vi "MotionController.vi"() -> (0 "error out":errorcluster)   [LabVIEW 2017]
uses:
  MCTypedef.ctl
  <vilib>/Instr/_visa.llb/VISA Configure Serial Port (Instr).vi
  <vilib>/Utility/inputDevices.llb/keyboardAcquire.vi
panel:
  in  "sp33d":dbl(knob)=0.5 step=0.5 scale=0.5..1.0
  in  "clear":bool
  out "read buffer":string
  in  "End Program":bool
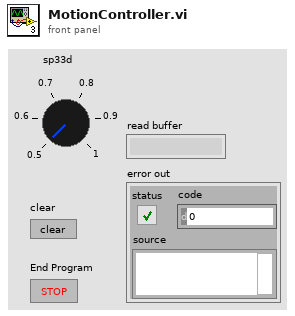
[diagram p1: front panel]
types:
  T1 = typedef "MCTypedef.ctl" = enum16{"idle", "forward", "reverse", "clear"}
  T2 = enum16{"0", "1", "2", "3", "4", "5", "6", "7", "8", "9", "A", "B", "C", "D", "E", "F", "G", "H", "I", "J", "K", "L", "M", "N", "O", "P", "Q", "R", "S", "T", "U", "V", "W", "X", "Y", "Z", "F1", "F2", "F3", "F4", "F5", "F6", "F7", "F8", "F9", "F10", "F11", "F12", "F13", "F14", "F15", "ADD", "BACK", "BACKSLASH", "CAPITAL", "COMMA", "DECIMAL", "DELETE", "DIVIDE", "DOWN", "END", "EQUALS", "ESCAPE", "GRAVE (`)", "HOME", "INSERT", "LBRACKET", "LCONTROL", "LEFT", "L ALT", "LSHIFT", "LWIN", "MINUS", "MULTIPLY", "NEXT", "NUMLOCK", "NUMPAD_0", "NUMPAD_1", "NUMPAD_2", "NUMPAD_3", "NUMPAD_4", "NUMPAD_5", "NUMPAD_6", "NUMPAD_7", "NUMPAD_8", "NUMPAD_9", "PAUSE", "PERIOD", "PRIOR (PG UP)", "RBRACKET", "RCONTROL", "RETURN", "RIGHT", "R ALT", "RSHIFT", "RWIN", "SCROLL", "SEMICOLON", "SLASH", "SPACE", "SUBTRACT", "TAB", "UP", "ENTER (num pad)", "' (quote)"}[]
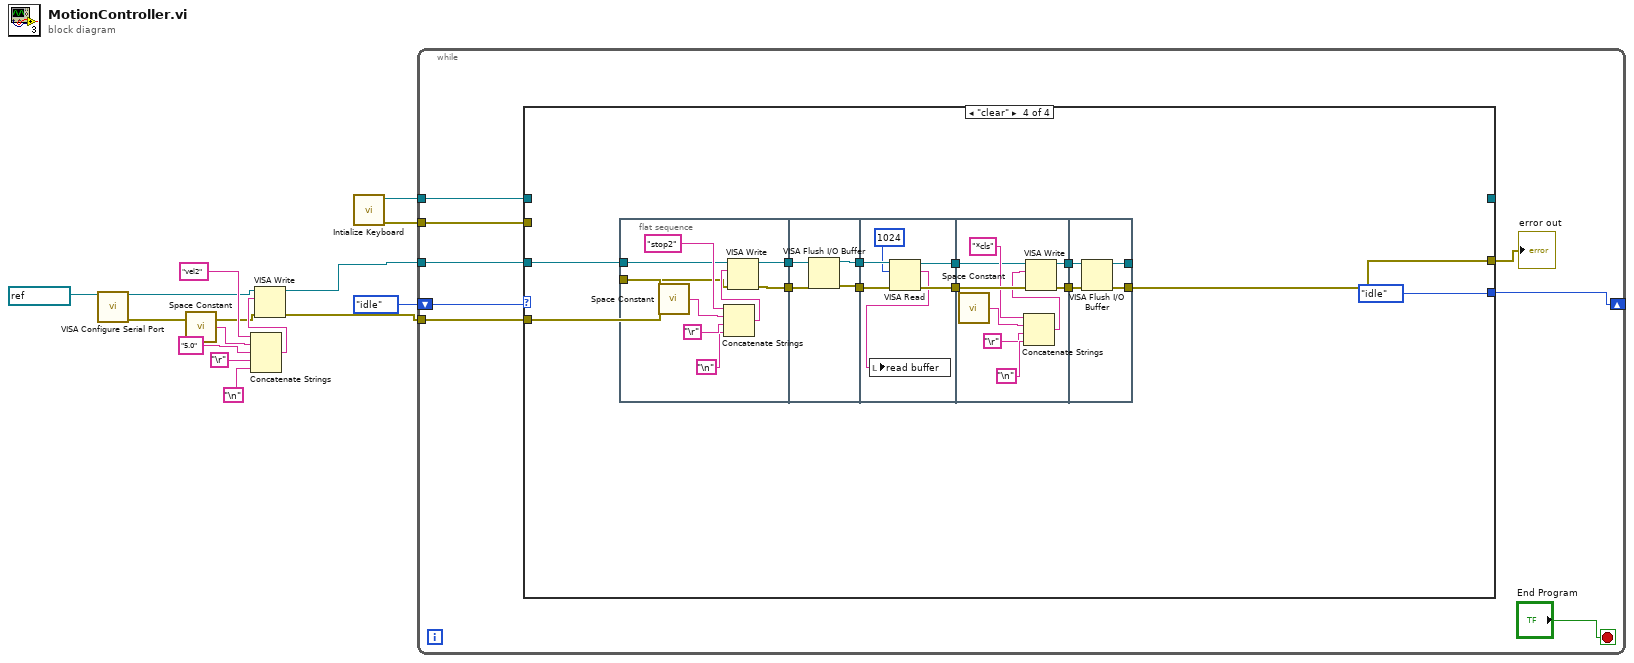
[diagram p0: block diagram]
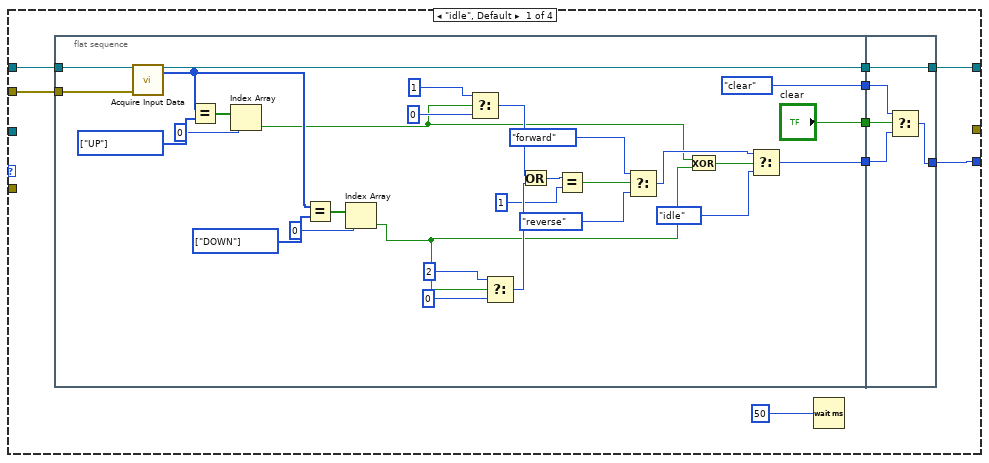
[diagram p2: hidden frame]
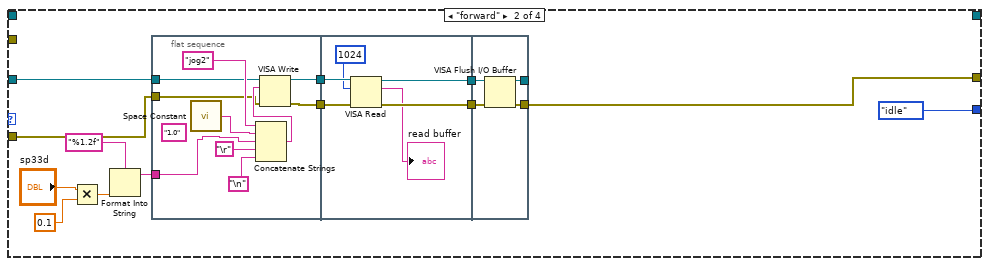
[diagram p3: hidden frame]
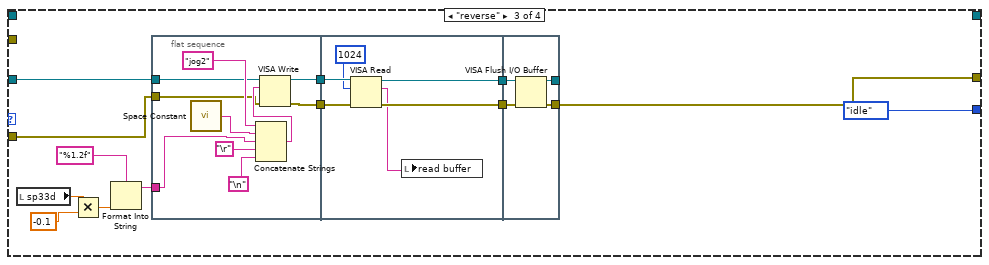
[diagram p4: hidden frame]
diagram:
  n1 = call-poly "VISA Configure Serial Port"("VISA resource name"=refnum<visa-resource-name> "COM1") -> ("VISA resource name out"=w5:refnum<visa-resource-name>, "error out"=w4:errorcluster)  [unwired: 13 in]
  n2 = call <vilib>:"Space Constant.vi"() -> ("String"=w11:string)
  n3 = Concatenate Strings("vel2" ("string"), w11, "5.0" ("string"), "\r", "\n") -> (w10:string)
  n4 = VISA Write(VISA resource name=w5, write buffer=w10, error in (no error)=w4) -> (VISA resource name out=w3:refnum<visa-resource-name>, error out=w2:errorcluster)  [unwired: 1 out]
  n5 = call <vilib>:"Intialize Keyboard.vi"() -> ("error out"=w12:errorcluster, "device ID"=w13:refnum<k1>)  [unwired: 10 in]
  n6 = while {
    shift-right: [w21] -> _
    shift-left: MCTypedef."idle" -> [w22]
    tunnel: w3 -> [w18]
    tunnel: w2 -> [w17]
    tunnel: w13 -> [w16]
    tunnel: w12 -> [w15]
    stop <- "End Program" stop-if-true
    n7 = case shown="\"clear\"" w22 {
      tunnel: [w23 MCTypedef."idle" MCTypedef."idle" MCTypedef."idle"] -> w21
      tunnel: [_ w73 w106 w142] -> w19
      tunnel: w18 -> [_ w72 w105 w141]
      tunnel: w17 -> [_ w71 w104 w140]
      tunnel: w16 -> [w30 _ _ _]
      tunnel: w15 -> [w28 _ _ _]
      tunnel: [w29 _ _ _] -> _
      frame "idle", Default {
        n8 = flat-sequence {
          tunnel: w30 -> [w46]
          tunnel: w28 -> [w41]
          tunnel: [w45] -> w27
          tunnel: [MCTypedef."clear" ("t")] -> w26
          tunnel: ["clear"] -> w25
          tunnel: [w32] -> w24
          tunnel: [w65] -> w29
          tunnel: w27 -> [w65]
          tunnel: w26 -> [w63]
          tunnel: w25 -> [w64]
          tunnel: w24 -> [w62]
          tunnel: [w61] -> w23
          frame #0 {
            w38 = T2 [enum."DOWN"] items=["0", "1", "2", "3", "4", "5", "6", "7", "8", "9", "A", "B", "C", "D", "E", "F", "G", "H", "I", "J", "K", "L", "M", "N", "O", "P", "Q", "R", "S", "T", "U", "V", "W", "X", "Y", "Z", "F1", "F2", "F3", "F4", "F5", "F6", "F7", "F8", "F9", "F10", "F11", "F12", "F13", "F14", "F15", "ADD", "BACK", "BACKSLASH", "CAPITAL", "COMMA", "DECIMAL", "DELETE", "DIVIDE", "DOWN", "END", "EQUALS", "ESCAPE", "GRAVE (`)", "HOME", "INSERT", "LBRACKET", "LCONTROL", "LEFT", "L ALT", "LSHIFT", "LWIN", "MINUS", "MULTIPLY", "NEXT", "NUMLOCK", "NUMPAD_0", "NUMPAD_1", "NUMPAD_2", "NUMPAD_3", "NUMPAD_4", "NUMPAD_5", "NUMPAD_6", "NUMPAD_7", "NUMPAD_8", "NUMPAD_9", "PAUSE", "PERIOD", "PRIOR (PG UP)", "RBRACKET", "RCONTROL", "RETURN", "RIGHT", "R ALT", "RSHIFT", "RWIN", "SCROLL", "SEMICOLON", "SLASH", "SPACE", "SUBTRACT", "TAB", "UP", "ENTER (num pad)", "' (quote)"] ("y")
            w44 = T2 [enum."UP"] items=["0", "1", "2", "3", "4", "5", "6", "7", "8", "9", "A", "B", "C", "D", "E", "F", "G", "H", "I", "J", "K", "L", "M", "N", "O", "P", "Q", "R", "S", "T", "U", "V", "W", "X", "Y", "Z", "F1", "F2", "F3", "F4", "F5", "F6", "F7", "F8", "F9", "F10", "F11", "F12", "F13", "F14", "F15", "ADD", "BACK", "BACKSLASH", "CAPITAL", "COMMA", "DECIMAL", "DELETE", "DIVIDE", "DOWN", "END", "EQUALS", "ESCAPE", "GRAVE (`)", "HOME", "INSERT", "LBRACKET", "LCONTROL", "LEFT", "L ALT", "LSHIFT", "LWIN", "MINUS", "MULTIPLY", "NEXT", "NUMLOCK", "NUMPAD_0", "NUMPAD_1", "NUMPAD_2", "NUMPAD_3", "NUMPAD_4", "NUMPAD_5", "NUMPAD_6", "NUMPAD_7", "NUMPAD_8", "NUMPAD_9", "PAUSE", "PERIOD", "PRIOR (PG UP)", "RBRACKET", "RCONTROL", "RETURN", "RIGHT", "R ALT", "RSHIFT", "RWIN", "SCROLL", "SEMICOLON", "SLASH", "SPACE", "SUBTRACT", "TAB", "UP", "ENTER (num pad)", "' (quote)"] ("y")
            n9 = call-poly <vilib>:"Acquire Input Data.vi"("device ID"=w46, "error in (no error)"=w41) -> ("device ID"=w45:refnum<k1>, "keys pressed"=w37:T2)  [unwired: 15 in, 1 out]
            n10 = Equal?(x=w37, y=w44) -> (x = y?=w43:bool[])
            n11 = Index Array(array=w43, index=0) -> (element=w36:bool)
            n12 = Equal?(x=w37, y=w38) -> (x = y?=w39:bool[])
            n13 = Index Array(array=w39, index=0) -> (element=w35:bool)
            n14 = Select(t=1, s=w36, f=0) -> (s? t:f=w55:i32)
            n15 = Select(t=2, s=w35, f=0) -> (s? t:f=w54:i32)
            n16 = Or(x=w55, y=w54) -> (x .or. y?=w53:i32)
            n17 = Equal?(x=w53, y=1) -> (x = y?=w51:bool)
            n18 = Select(t=MCTypedef."forward", s=w51, f=MCTypedef."reverse") -> (s? t:f=w47:T1)
            n19 = Exclusive Or(1:w35, 2:w36) -> (0:w60:bool)
            n20 = Select(t=w47, s=w60, f=MCTypedef."idle") -> (s? t:f=w32:T1)
          }
          frame #1 {
            n21 = Select(t=w63, s=w64, f=w62) -> (s? t:f=w61:T1)
          }
        }
        n22 = Wait (ms)(milliseconds to wait=u32 50) -> ()  [unwired: 1 out]
      }
      frame "forward" {
        n23 = Multiply(x="sp33d", y=0.1) -> (x*y=w68:dbl)
        n24 = Format Into String(format string="%1.2f", w68) -> (resulting string=w66:string)  [unwired: 2 in, 1 out]
        n25 = flat-sequence {
          tunnel: [w88] -> w78
          tunnel: [w87] -> w77
          tunnel: w72 -> [w81]
          tunnel: w71 -> [w80]
          tunnel: w66 -> [w79]
          tunnel: w78 -> [w94]
          tunnel: w77 -> [w93]
          tunnel: [w92] -> w76
          tunnel: [w91] -> w75
          tunnel: w76 -> [w97]
          tunnel: w75 -> [w98]
          tunnel: [w96] -> _
          tunnel: [w95] -> w73
          frame #0 {
            (unwired) "1.0" ("string")
            n26 = call <vilib>:"Space Constant.vi"() -> ("String"=w82:string)
            n27 = Concatenate Strings("jog2" ("string"), w82, w79, "\r", "\n") -> (w83:string)
            n28 = VISA Write(VISA resource name=w81, write buffer=w83, error in (no error)=w80) -> (VISA resource name out=w88:refnum<visa-resource-name>, error out=w87:errorcluster)  [unwired: 1 out]
          }
          frame #1 {
            n29 = VISA Read(VISA resource name=w94, byte count=u32 1024, error in (no error)=w93) -> (VISA resource name out=w92:refnum<visa-resource-name>, read buffer=→"read buffer":string, error out=w91:errorcluster)  [unwired: 1 out]
          }
          frame #2 {
            n30 = VISA Flush I/O Buffer(VISA resource name=w97, error in (no error)=w98) -> (VISA resource name out=w96:refnum<visa-resource-name>, error out=w95:errorcluster)  [unwired: 1 in]
          }
        }
      }
      frame "reverse" {
        n31 = local read "sp33d"() -> (w100:dbl)
        n32 = Multiply(x=w100, y=-0.1) -> (x*y=w103:dbl)
        n33 = Format Into String(format string="%1.2f", w103) -> (resulting string=w99:string)  [unwired: 2 in, 1 out]
        n34 = flat-sequence {
          tunnel: [w121] -> w111
          tunnel: [w120] -> w110
          tunnel: w105 -> [w114]
          tunnel: w104 -> [w113]
          tunnel: w99 -> [w112]
          tunnel: w111 -> [w127]
          tunnel: w110 -> [w126]
          tunnel: [w125] -> w109
          tunnel: [w124] -> w108
          tunnel: w109 -> [w130]
          tunnel: w108 -> [w131]
          tunnel: [w129] -> _
          tunnel: [w128] -> w106
          frame #0 {
            n35 = call <vilib>:"Space Constant.vi"() -> ("String"=w115:string)
            n36 = Concatenate Strings("jog2" ("string"), w115, w112, "\r", "\n") -> (w116:string)
            n37 = VISA Write(VISA resource name=w114, write buffer=w116, error in (no error)=w113) -> (VISA resource name out=w121:refnum<visa-resource-name>, error out=w120:errorcluster)  [unwired: 1 out]
          }
          frame #1 {
            n38 = VISA Read(VISA resource name=w127, byte count=u32 1024, error in (no error)=w126) -> (VISA resource name out=w125:refnum<visa-resource-name>, read buffer=w122:string, error out=w124:errorcluster)  [unwired: 1 out]
            n39 = local write "read buffer"(w122) -> ()
          }
          frame #2 {
            n40 = VISA Flush I/O Buffer(VISA resource name=w130, error in (no error)=w131) -> (VISA resource name out=w129:refnum<visa-resource-name>, error out=w128:errorcluster)  [unwired: 1 in]
          }
        }
      }
      frame "clear" {
        n41 = flat-sequence {
          tunnel: [w152] -> w135
          tunnel: [w151] -> w133
          tunnel: w141 -> [w147]
          tunnel: w140 -> [w146]
          tunnel: w135 -> [w156]
          tunnel: [w154] -> w134
          tunnel: w133 -> [w155]
          tunnel: [w153] -> w132
          tunnel: w134 -> [w162]
          tunnel: w132 -> [w161]
          tunnel: [w160] -> w138
          tunnel: [w157] -> w136
          tunnel: [w171] -> w139
          tunnel: w138 -> [w170]
          tunnel: [w169] -> w137
          tunnel: w136 -> [w163]
          tunnel: w139 -> [w174]
          tunnel: w137 -> [w175]
          tunnel: [w173] -> _
          tunnel: [w172] -> w142
          frame #0 {
            n42 = call <vilib>:"Space Constant.vi"() -> ("String"=w148:string)
            n43 = Concatenate Strings("stop2" ("string"), w148, "\r", "\n") -> (w149:string)
            n44 = VISA Write(VISA resource name=w147, write buffer=w149, error in (no error)=w146) -> (VISA resource name out=w152:refnum<visa-resource-name>, error out=w151:errorcluster)  [unwired: 1 out]
          }
          frame #1 {
            n45 = VISA Flush I/O Buffer(VISA resource name=w156, error in (no error)=w155) -> (VISA resource name out=w154:refnum<visa-resource-name>, error out=w153:errorcluster)  [unwired: 1 in]
          }
          frame #2 {
            n46 = VISA Read(VISA resource name=w162, byte count=u32 1024, error in (no error)=w161) -> (VISA resource name out=w157:refnum<visa-resource-name>, read buffer=w158:string, error out=w160:errorcluster)  [unwired: 1 out]
            n47 = local write "read buffer"(w158) -> ()
          }
          frame #3 {
            n48 = call <vilib>:"Space Constant.vi"() -> ("String"=w166:string)
            n49 = Concatenate Strings("*cls" ("string"), w166, "\r", "\n") -> (w164:string)
            n50 = VISA Write(VISA resource name=w163, write buffer=w164, error in (no error)=w170) -> (VISA resource name out=w171:refnum<visa-resource-name>, error out=w169:errorcluster)  [unwired: 1 out]
          }
          frame #4 {
            n51 = VISA Flush I/O Buffer(VISA resource name=w174, error in (no error)=w175) -> (VISA resource name out=w173:refnum<visa-resource-name>, error out=w172:errorcluster)  [unwired: 1 in]
          }
        }
      }
    }
    "error out" <- w19
  }
